vi "pp_trialTypes_selectType.vi"(10 "Trial Type":enum16{"OFF", "GO", "NOGO", "TEST"}(ring)=enum."GO", 11 "Trial Types":T1(array[cluster]) {"Stim P2" min=0.0; "Trial Weight" step=1; "Stim P1" min=0.0; "Stim Dur (s)" min=0.0; "Trial Code" min=1 step=1}) -> (0 "Number of Selected Trial Types":i32, 1 "Weight sums":i32, 3 "Selected Trial Types":T1(array[cluster]) {"Stim P2" min=0.0; "Trial Weight" step=1; "Stim P1" min=0.0; "Stim Dur (s)" min=0.0; "Trial Code" min=1 step=1})   [LabVIEW 2013]
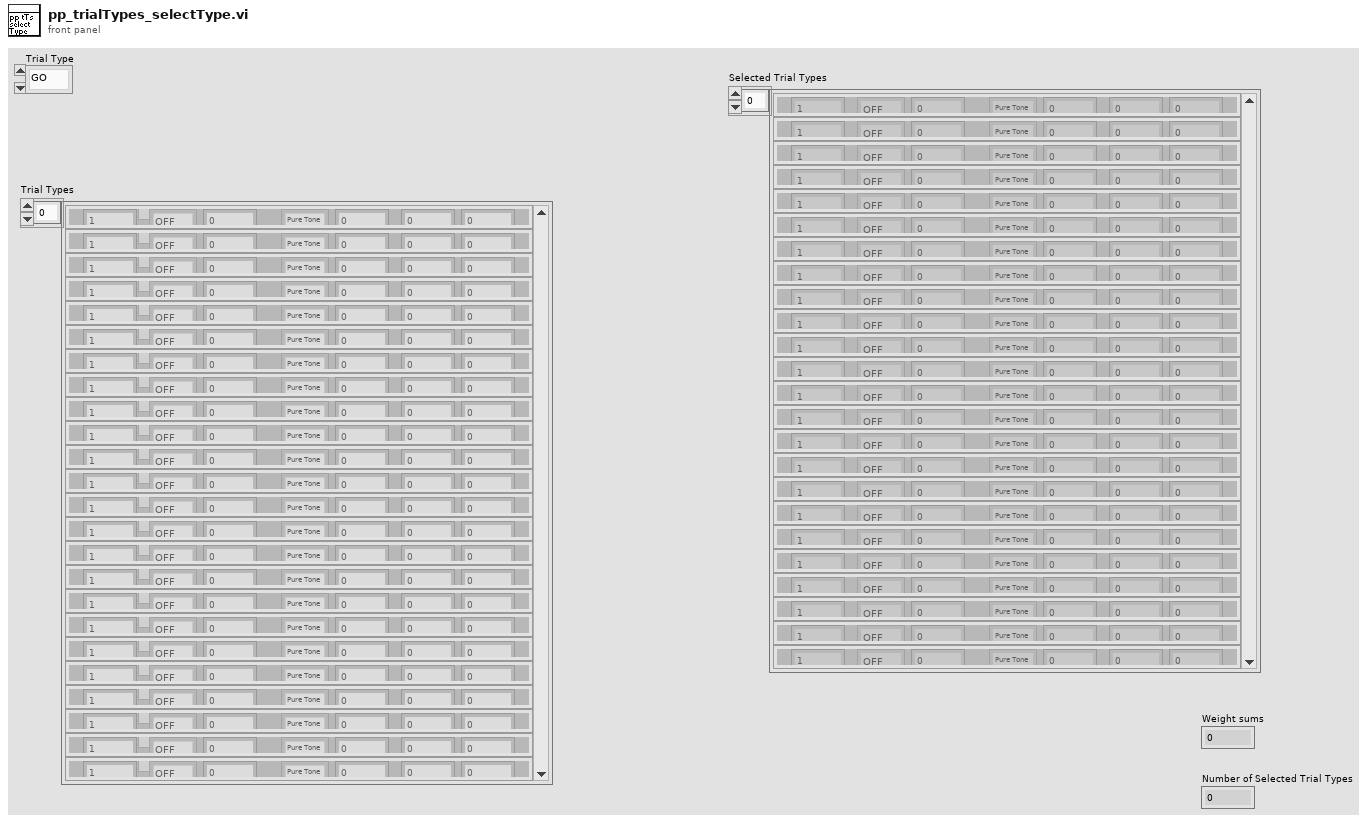
[diagram p1: front panel]
types:
  T1 = cluster{"Trial Code":u16, "Trial Type":enum16{"OFF", "GO", "NOGO", "TEST"}, "Trial Weight":u32, "Stim Type":enum16{"Pure Tone", "FM Sweep"}, "Stim Dur (s)":dbl, "Stim P1":dbl, "Stim P2":dbl}[]
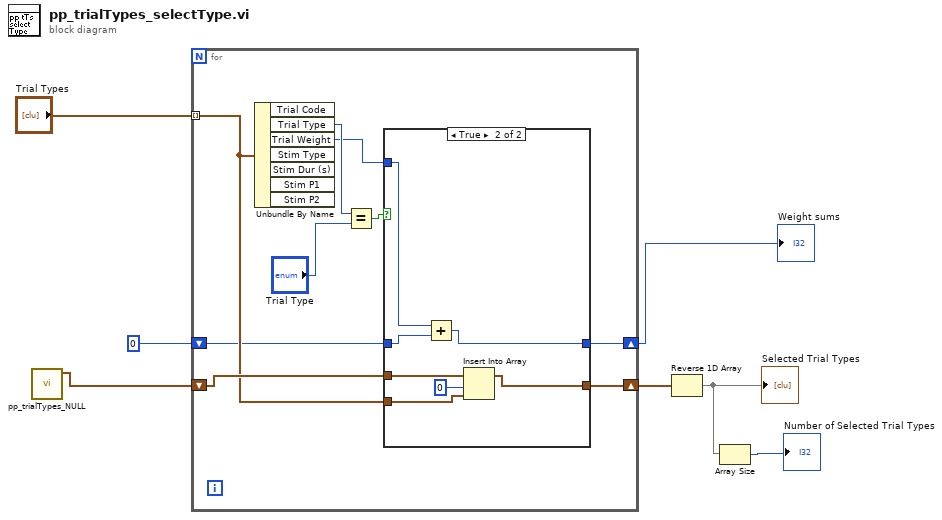
[diagram p0: block diagram]
diagram:
  n1 = call "pp_trialTypes_NULL.vi"() -> ("Trial Types Null"=w1:T1)  [unwired: 10 in, 1 out]
  n2 = for {
    tunnel: "Trial Types" -> [w11] mode=indexing
    shift-right: [w12] -> w6
    shift-left: w1 -> [w13]
    shift-right: [w9] -> w2
    shift-left: 0 ("Weight sums") -> [w10]
    n3 = Unbundle By Name(w11) -> ("Trial Type"=w16:enum16{"OFF", "GO", "NOGO", "TEST"}, "Trial Weight"=w8:u32)  [unwired: 5 out]
    n4 = Equal?(x=w16, y="Trial Type") -> (x = y?=w14:bool)
    n5 = case shown="True" w14 {
      tunnel: w13 -> [w18 w25]
      tunnel: [w18 w24] -> w12
      tunnel: w11 -> [_ w22]
      tunnel: w10 -> [w17 w21]
      tunnel: [w17 w19] -> w9
      tunnel: w8 -> [_ w20]
      frame False {
      }
      frame True {
        n6 = Add(x=w20, y=w21) -> (x+y=w19:u32)
        n7 = Insert Into Array(array=w25, index=0, new element=w22) -> (w24:T1)
      }
    }
  }
  "Weight sums" <- w2
  n8 = Reverse 1D Array(array=w6) -> (reversed array=w5:T1)
  "Selected Trial Types" <- w5
  n9 = Array Size(array=w5) -> (size(s)=→"Number of Selected Trial Types":i32)
